vi "Triggers logic.vi"(0 "Imaging Protocol":T6=enum."Live Imaging", 1 "PXI Trigger Enable":T7, 3 "General trig. pulse width":T1={"Trigger 1 function"=enum."Line trigger", "Pulse width (ticks)-Line Trig."=80000, "Pulse width (ticks)-Frame/Cycle Trig."=80, "Pulse width (ticks)-Trial trig."=80, "Pulse width (ticks)-Start of Exp. trig."=80000}, 4 "Stimulus Trigger Setup":T5={"Trigger period in live protocols (80MHz Cycles)"=800000000, "Pulse width in live protocols (80MHz Cycles)"=40000000, "Enable stimulus in live protocols"=FALSE, "Trigger delay in funct. protocols (80MHz Cycles)"=0, "Pulse width in funct. protocols (80MHz Cycles)"=400000, "Enable stimulus in funct. protocols"=FALSE}, 5 "Encored_trigger OR Line_signal":bool, 6 "live_scan":bool, 7 "Ctr_trig_signal":bool, 9 "Trial_signal":bool, 10 "Experiment start":bool, 11 "Start_acq_signal":bool, 12 "Abort triggers":bool, 13 "FPGA state":T3=enum."Wait N after Trigger") -> (15 "Triggers output cluster":T4)   [LabVIEW 2020]
uses:
  FPGA Typedefs/Inter-loop signals.ctl
  Typedefs/Imaging Protocols enum.ctl
  FPGA Typedefs/PXI Trigger Enable cluster.ctl
  FPGA Typedefs/Stimulus trigger delays cluster.ctl
  FPGA Typedefs/Triggers output cluster.ctl
  FPGA Typedefs/Image State.ctl
  FPGA Typedefs/General trig pulse width.ctl
  Typedefs/Trigger 1 selector enum.ctl
panel:
  # "(80=1us)"
  # "(80=1us)"
  # "(80000=1ms)"
  # "(80000=1ms)"
  # "Limited to 53.5 sec (if U32)"
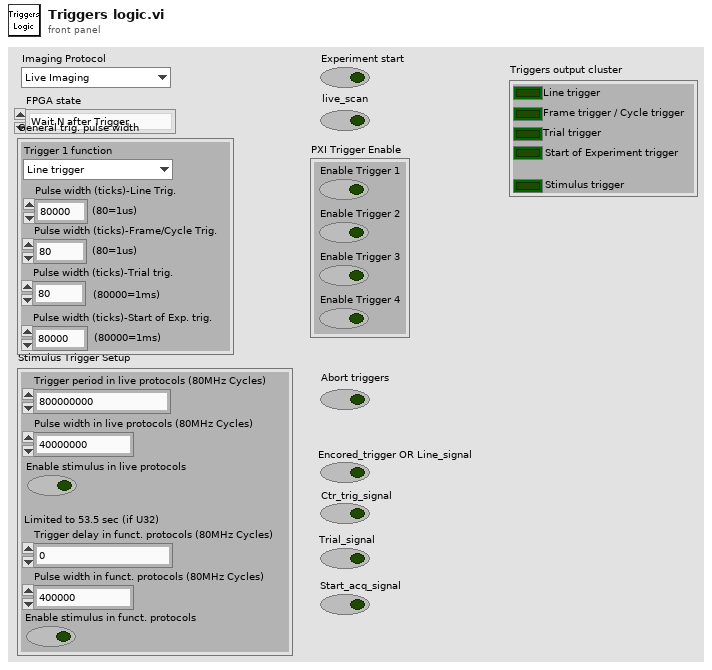
[diagram p1: front panel]
types:
  T1 = typedef "General trig pulse width.ctl" = cluster{"Trigger 1 function":T2, "Pulse width (ticks)-Line Trig.":u32, "Pulse width (ticks)-Frame/Cycle Trig.":u32, "Pulse width (ticks)-Trial trig.":u32, "Pulse width (ticks)-Start of Exp. trig.":u32}
  T2 = typedef "Trigger 1 selector enum.ctl" = enum16{"Encoder trigger", "Line trigger", "Control system's ref frame acknowledgement"}
  T3 = typedef "Image State.ctl" = enum16{"Start Up", "Wait for Trigger", "Wait N after Trigger", "DAQ Pointing", "DAQ Scan", "Reference Scan", "Pointing AOL Fill", "Scan AOL FILL", "Reference AOL Fill"}
  T4 = typedef "Triggers output cluster.ctl" = cluster{"Line trigger":bool, "Frame trigger / Cycle trigger":bool, "Trial trigger":bool, "Start of Experiment trigger":bool, "Stimulus trigger":bool}
  T5 = typedef "Stimulus trigger delays cluster.ctl" = cluster{"Trigger period in live protocols (80MHz Cycles)":u32, "Pulse width in live protocols (80MHz Cycles)":u32, "Enable stimulus in live protocols":bool, "Trigger delay in funct. protocols (80MHz Cycles)":u32, "Pulse width in funct. protocols (80MHz Cycles)":u32, "Enable stimulus in funct. protocols":bool}
  T6 = typedef "Imaging Protocols enum.ctl" = enum16{"AOL Z-Stack", "Motor Z Stack", "Functional Acquisition", "Single Plane Acquisition", "Volume Acquisition", "Live Imaging", "Live Plane Imaging", "Live Volume Imaging"}
  T7 = typedef "PXI Trigger Enable cluster.ctl" = cluster{"Enable Trigger 1":bool, "Enable Trigger 2":bool, "Enable Trigger 3":bool, "Enable Trigger 4":bool}
  T8 = typedef "Inter-loop signals.ctl" = cluster{"Encored_trigger OR Line_signal":bool, "Ctr_trig_signal":bool, "Trial_signal":bool, "Start_acq_signal":bool}
  T9 = typedef "PXI Trigger lines value cluster.ctl" = cluster{"Value of Trigger 1":bool, "Value of Trigger 2":bool, "Value of Trigger 3":bool, "Value of Trigger 4":bool, "Value of Trigger 5":bool}
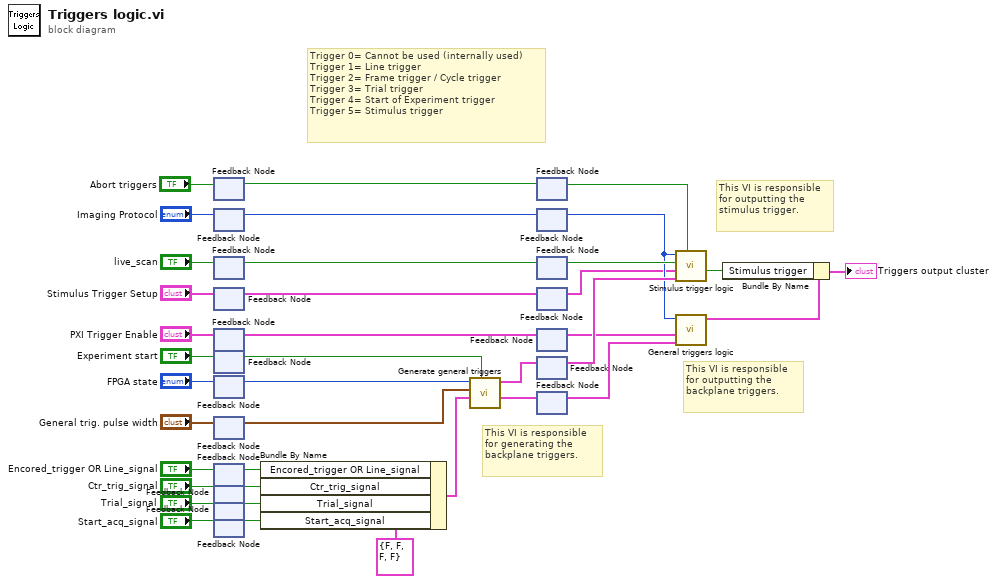
[diagram p0: block diagram]
diagram:
  # "This VI is responsible for generating the  backplane triggers."
  # "This VI is responsible for outputting the  stimulus trigger."
  # "Trigger 0= Cannot be used (internally used)\nTrigger 1= Line trigger\nTrigger 2= Frame trigger / Cycle trigger\nTrigger 3= Trial trigger\nTrigger 4= Start of Experiment trigger\nTrigger 5= Stimulus trigger"
  # "This VI is responsible for outputting the  backplane triggers."
  n1 = feedback #1() -> (w1:bool)  [unwired: 1 in]
  n2 = feedback-in #1("Abort triggers") -> ()
  n3 = feedback #2() -> (w6:T6)  [unwired: 1 in]
  n4 = feedback-in #2("Imaging Protocol") -> ()
  n5 = feedback #3() -> (w12:bool)  [unwired: 1 in]
  n6 = feedback-in #3("live_scan") -> ()
  n7 = feedback #4() -> (w5:T5)  [unwired: 1 in]
  n8 = feedback-in #4("Stimulus Trigger Setup") -> ()
  n9 = feedback #5() -> (w4:T7)  [unwired: 1 in]
  n10 = feedback-in #5("PXI Trigger Enable") -> ()
  n11 = feedback #6() -> (w3:bool)  [unwired: 1 in]
  n12 = feedback-in #6("Experiment start") -> ()
  n13 = feedback #7() -> (w11:T3)  [unwired: 1 in]
  n14 = feedback-in #7("FPGA state") -> ()
  n15 = feedback #8() -> (w2:T1)  [unwired: 1 in]
  n16 = feedback-in #8("General trig. pulse width") -> ()
  n17 = feedback #9() -> (w10:bool)  [unwired: 1 in]
  n18 = feedback-in #9("Encored_trigger OR Line_signal") -> ()
  n19 = feedback #10() -> (w9:bool)  [unwired: 1 in]
  n20 = feedback-in #10("Ctr_trig_signal") -> ()
  n21 = feedback #11() -> (w8:bool)  [unwired: 1 in]
  n22 = feedback-in #11("Trial_signal") -> ()
  n23 = feedback #12() -> (w7:bool)  [unwired: 1 in]
  n24 = feedback-in #12("Start_acq_signal") -> ()
  n25 = Bundle By Name(cluster=T8 {"Encored_trigger OR Line_signal"=FALSE, "Ctr_trig_signal"=FALSE, "Trial_signal"=FALSE, "Start_acq_signal"=FALSE} ("Inter-loop signals"), "Encored_trigger OR Line_signal"=w10, "Ctr_trig_signal"=w9, "Trial_signal"=w8, "Start_acq_signal"=w7) -> (w15:T8)
  n26 = call "Generate general triggers.vi"("Experiment start"=w3, "Inter-loop signals"=w15, "General trig. pulse width"=w2, "FPGA state"=w11) -> ("Trigger lines value"=w14:T9, "Unmodified signal values"=w13:T9)  [unwired: 6 in]
  n27 = feedback #13() -> (w17:bool)  [unwired: 1 in]
  n28 = feedback-in #13(w1) -> ()
  n29 = feedback #14() -> (w24:T6)  [unwired: 1 in]
  n30 = feedback-in #14(w6) -> ()
  n31 = feedback #15() -> (w30:bool)  [unwired: 1 in]
  n32 = feedback-in #15(w12) -> ()
  n33 = feedback #16() -> (w21:T5)  [unwired: 1 in]
  n34 = feedback-in #16(w5) -> ()
  n35 = feedback #17() -> (w19:T7)  [unwired: 1 in]
  n36 = feedback-in #17(w4) -> ()
  n37 = feedback #18() -> (w32:T9)  [unwired: 1 in]
  n38 = feedback-in #18(w13) -> ()
  n39 = feedback #19() -> (w33:T9)  [unwired: 1 in]
  n40 = feedback-in #19(w14) -> ()
  n41 = call "Stimulus trigger logic.vi"("Abort triggers"=w17, "Unmodified signal values"=w32, "Stimulus Trigger Setup"=w21, "live_scan"=w30, "Imaging Protocol"=w24) -> ("Stimulus trigger"=w36:bool)  [unwired: 6 in]
  n42 = call "General triggers logic.vi"("Trigger lines value"=w33, "PXI Trigger Enable"=w19, "Imaging Protocol"=w24) -> ("Triggers output cluster"=w38:T4)  [unwired: 8 in]
  n43 = Bundle By Name(cluster=w38, "Stimulus trigger"=w36) -> (→"Triggers output cluster":T4)
